vi "LSCI332 SetZoneInfo.vi"(0 "VISA Rsrc":refnum<visa-resource-name>="GPIB0::12::INSTR", 5 "Boucle(1)":u32(ring) caption="Boucle" items=["Boucle 1", "Boucle 2"], 7 "Zone":u32=1 min=1 max=10 step=1, 9 "Paramètres":T1={"TempFin"=400.0, "P"=1000.0, "I"=0.0, "D"=0, "ManualOutput(%)"=0.0, "Range"=5} {"D" max=200 step=1; "I" min=0.0 max=1000.0 step=0.1 format="%#.1f"; "Range" max=3 step=1; "ManualOutput(%)" min=-100.0 max=100.0 step=0.01 format="%#.2g"; "P" min=0.0 max=1000.0 step=0.1 format="%#.1f"; "TempFin" min=0.0 max=400.0 step=0.001 format="%#.3g"}, 11 "error in (no error)":errorcluster) -> (15 "error out":errorcluster)   [LabVIEW 2012]
doc: "Ce VI écrit les paramètres de la zone de contrôle spécifiée dans le contrôlleur"
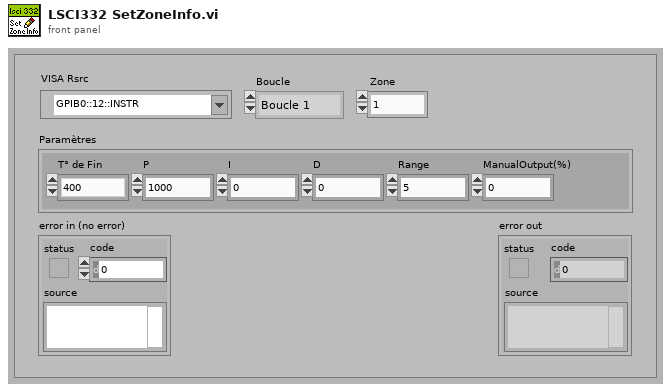
[diagram p1: front panel]
types:
  T1 = cluster{"TempFin":dbl, "P":dbl, "I":dbl, "D":u32, "ManualOutput(%)":dbl, "Range":u32}
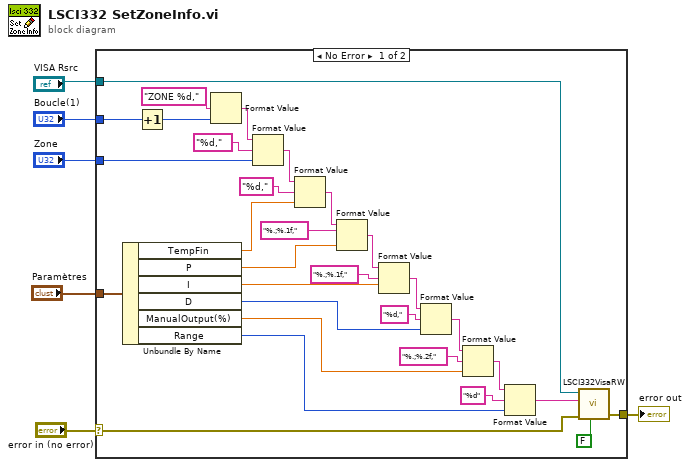
[diagram p0: block diagram]
diagram:
  n1 = case shown="No Error" "error in (no error)" {
    selector: "error in (no error)" -> [w8 w37]
    tunnel: "VISA Rsrc" -> [w36 _]
    tunnel: "Boucle(1)" -> [w34 _]
    tunnel: "Zone" -> [w24 _]
    tunnel: [w35 w37] -> w3
    tunnel: "Paramètres" -> [w23 _]
    frame No Error {
      n2 = Unbundle By Name(w23) -> ("TempFin"=w22:dbl, "P"=w21:dbl, "I"=w20:dbl, "D"=w19:u32, "ManualOutput(%)"=w17:dbl, "Range"=w18:u32)
      n3 = Increment(x=w34) -> (x+1=w25:u32)
      n4 = Format Value(format string="ZONE %d,", value (0)=w25) -> (output string=w12:string)  [unwired: 1 in]
      n5 = Format Value(string ("")=w12, format string="%d,", value (0)=w24) -> (output string=w11:string)
      n6 = Format Value(string ("")=w11, format string="%d,", value (0)=w22) -> (output string=w29:string)
      n7 = Format Value(string ("")=w29, format string="%.;%.1f,", value (0)=w21) -> (output string=w28:string)
      n8 = Format Value(string ("")=w28, format string="%.;%.1f,", value (0)=w20) -> (output string=w27:string)
      n9 = Format Value(string ("")=w27, format string="%d,", value (0)=w19) -> (output string=w26:string)
      n10 = Format Value(string ("")=w26, format string="%.;%.2f,", value (0)=w17) -> (output string=w10:string)
      n11 = Format Value(string ("")=w10, format string="%d", value (0)=w18) -> (output string=w9:string)
      n12 = call <userlib>:"LSCI332VisaRW.vi"("Lecture?(T)"=FALSE, "error in (no error)"=w8, "ChaineCom"=w9, "VISA Rsrc"=w36) -> ("error out"=w35:errorcluster)  [unwired: 3 in, 3 out]
    }
    frame Error {
    }
  }
  "error out" <- w3
